vi "Kalman Filter - Predict Step.vi"(8 "Dynamical System Matrices In":T1, 9 "Control Input":T2, 10 "Initial Covariance":T2, 11 "Initial State":T2) -> (0 "Dynamical System Matrices Out":T1, 2 "Predicted Covariance":T2, 3 "Predicted State":T2)   [LabVIEW 2020]
uses:
  <vilib>/Analysis/Matrix/Datatypes/RealMatrix.ctl
  ctl/Dynamical System Matrices.ctl
  <vilib>/Analysis/Matrix/NI_Matrix.lvlib
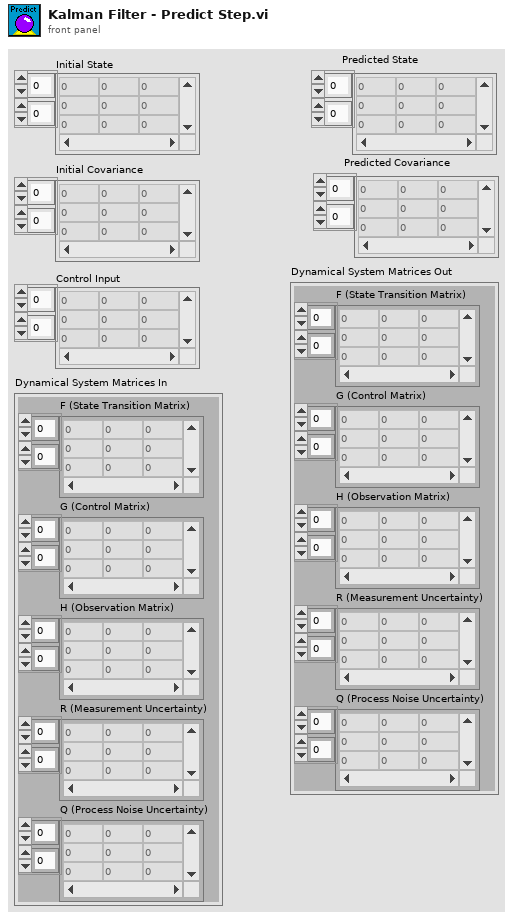
[diagram p1: front panel]
types:
  T1 = typedef "Dynamical System Matrices.ctl" = cluster{"F (State Transition Matrix)":T2, "G (Control Matrix)":T2, "H (Observation Matrix)":T2, "R (Measurement Uncertainty)":T2, "Q (Process Noise Uncertainty)":T2}
  T2 = typedef "NI_Matrix.lvlib/RealMatrix.ctl" = dbl[][]
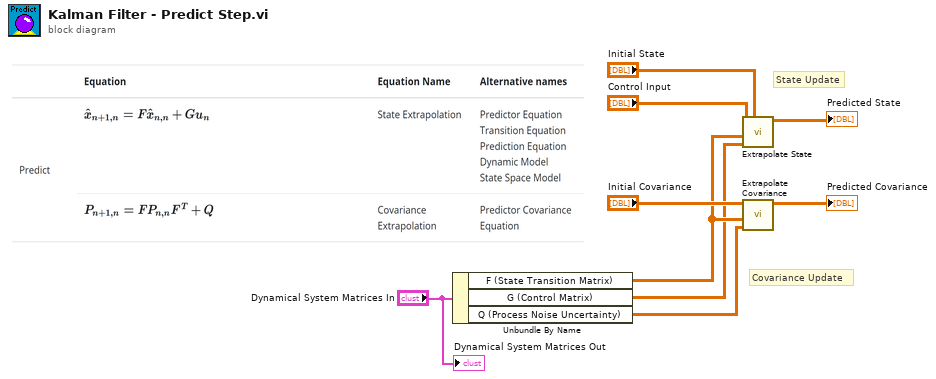
[diagram p0: block diagram]
diagram:
  # "Covariance Update"
  # "State Update"
  n1 = Unbundle By Name("Dynamical System Matrices In") -> ("F (State Transition Matrix)"=w4:T2, "G (Control Matrix)"=w2:T2, "Q (Process Noise Uncertainty)"=w3:T2)
  n2 = call "Extrapolate State.vi"("Initial State"="Initial State", "G"=w2, "F"=w4, "Control"="Control Input") -> ("Predicted State"=→"Predicted State":T2)  [unwired: 7 in]
  n3 = call "Extrapolate Covariance.vi"("Q"=w3, "F"=w4, "Covariance"="Initial Covariance") -> ("Predicted Covariance"=→"Predicted Covariance":T2)  [unwired: 8 in]
  "Dynamical System Matrices Out" <- "Dynamical System Matrices In"
